vi "ex_readSimpleFile.vi"(5 "first time":bool, 6 "Path":path, 7 "number of lines (all:-1)":i32=-1, 8 "error in":errorcluster, 9 "Generic Header In":string[](array[string]), 10 "string in":string, 11 "Generic Params":T2) -> (0 "error out":errorcluster, 1 "Generic Header Out":string[](array[string]), 2 "string remainder":string, 3 "Signals":waveform(dbl)[](array[waveform]), 4 "EOF":bool)   [LabVIEW 2020]
uses:
  <vilib>/express/express input/ExFileReadBlock.llb/ex_ReadFileGenericParams.ctl
  <vilib>/express/express shared/transition.llb/ex_WaveformAttribs.ctl
  <vilib>/express/express shared/transition.llb/Build Exp Wvfrm (Wvfrm).vi
panel:
  in  "Express Waveform Attributes":T1 {"Timestamp" format="%<%X\n%x>T"; "Start Timestamp" format="%<%X\n%x>T"}
  in  "Array":string[](array[string])
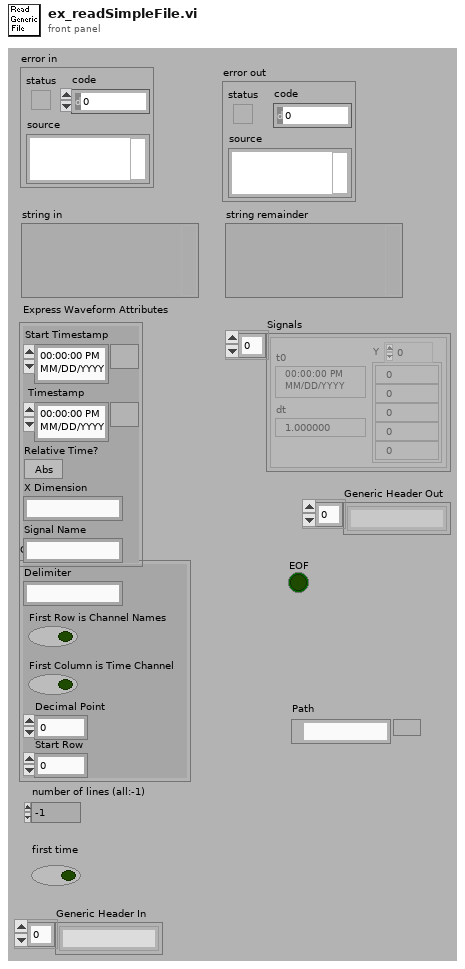
[diagram p1: front panel]
types:
  T1 = typedef "ex_WaveformAttribs.ctl" = cluster{"Start Timestamp":timestamp, "Timestamp":timestamp, "Relative Time?":bool, "X Dimension":string, "Signal Name":string}
  T2 = typedef "ex_ReadFileGenericParams.ctl" = cluster{"Delimiter":string, "First Row is Channel Names":bool, "First Column is Time Channel":bool, "Decimal Point":i32, "Start Row":i32}
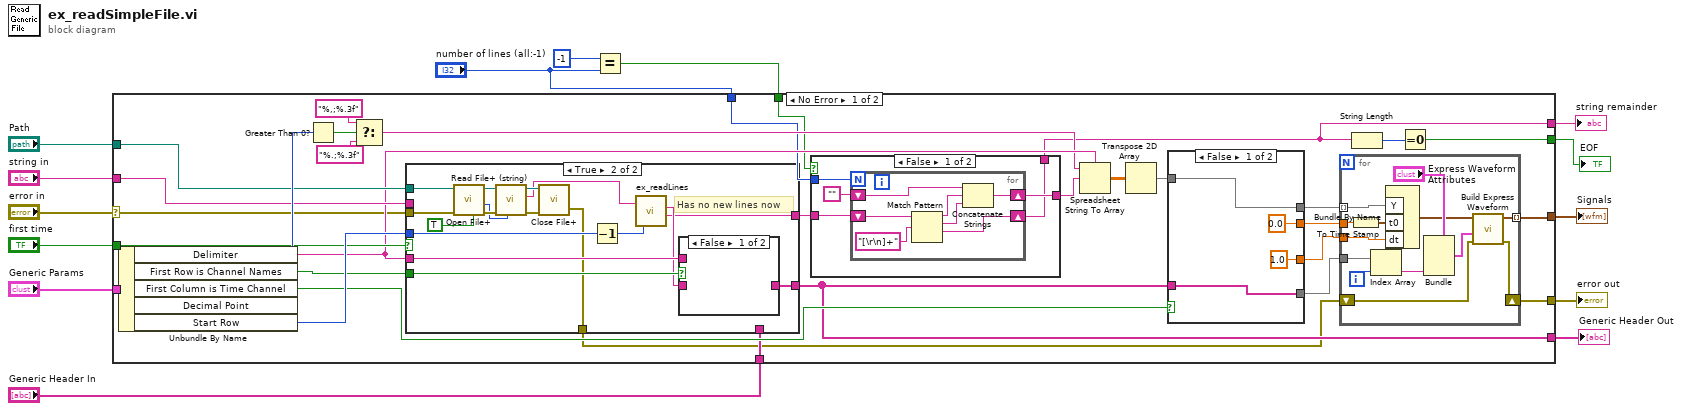
[diagram p0: block diagram]
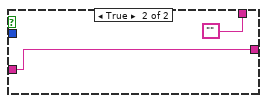
[diagram p2: hidden frame]
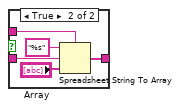
[diagram p5: hidden frame]
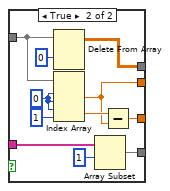
[diagram p6: hidden frame]
diagram:
  n1 = Equal?(x=-1 ("y"), y="number of lines (all:-1)") -> (x = y?=w5:bool)
  n2 = case shown="No Error" "error in" {
    selector: "error in" -> [w16 w117]
    tunnel: [w31 w117] -> w14
    tunnel: [w46 _] -> w13
    tunnel: "Generic Params" -> [w45 _]
    tunnel: "string in" -> [w32 _]
    tunnel: "first time" -> [w30 _]
    tunnel: [w29 _] -> w8
    tunnel: "Generic Header In" -> [w28 _]
    tunnel: [w17 _] -> w6
    tunnel: w5 -> [w20 _]
    tunnel: "number of lines (all:-1)" -> [w21 _]
    tunnel: [w26 _] -> w2
    tunnel: "Path" -> [w25 _]
    frame No Error {
      n3 = Unbundle By Name(w45) -> ("Delimiter"=w23:string, "First Row is Channel Names"=w42:bool, "First Column is Time Channel"=w41:bool, "Decimal Point"=w44:i32, "Start Row"=w43:i32)
      n4 = Greater Than 0?(x=w44) -> (x > 0?=w38:bool)
      n5 = Select(t="%,;%.3f" ("format (%.3f)"), s=w38, f="%.;%.3f" ("format (%.3f)")) -> (s? t:f=w22:string)
      n6 = case shown="True" w30 {
        tunnel: w23 -> [_ w83]
        tunnel: w43 -> [_ w82]
        tunnel: w42 -> [w64 w81]
        tunnel: [w65 w79] -> w19
        tunnel: [w63 w78] -> w29
        tunnel: w32 -> [w65 _]
        tunnel: w28 -> [w62 _]
        tunnel: w25 -> [_ w72]
        tunnel: w16 -> [w61 w68]
        tunnel: [w61 w67] -> w15
        frame False {
          n7 = case shown="False" w64 {
            tunnel: [_ w66] -> w63
            tunnel: w62 -> [_ w66]
            frame False {
            }
            frame True {
            }
          }
        }
        frame True {
          # "Has no new lines now"
          n8 = call <vilib>:"Open File+.vi"("advisory dialog? (display:T)"=TRUE, "error in (not an error)"=w68, "file path (\" \")"=w72) -> ("error out"=w73:errorcluster, "file size (bytes)"=w70:i32, "refnum"=w75:refnum<file>)  [unwired: 4 in, 2 out]
          n9 = call <vilib>:"Read File+ (string).vi"("count"=w70, "error in (no error)"=w73, "refnum"=w75) -> ("error out"=w74:errorcluster, "string"=w71:string, "dup refnum"=w76:refnum<file>)  [unwired: 2 in, 4 out]
          n10 = call <vilib>:"Close File+.vi"("error in (no error)"=w74, "refnum"=w76) -> ("error out"=w67:errorcluster)  [unwired: 5 out]
          n11 = Decrement(x=w82) -> (x-1=w77:i32)
          n12 = call <vilib>:"ex_readLines.vi"("line string"=w71, "# Lines to Skip"=w77) -> ("Channel Names"=w80:string, "Data"=w79:string)  [unwired: 2 out]
          n13 = case shown="False" w81 {
            tunnel: w80 -> [_ w88]
            tunnel: w83 -> [_ w86]
            tunnel: [_ w84] -> w78
            frame False {
            }
            frame True {
              n14 = Spreadsheet String To Array(delimiter (Tab)=w86, format string="%s", spreadsheet string=w88, array type (2D Dbl)="Array") -> (array=w84:string[])
            }
          }
        }
      }
      n15 = case shown="False" w20 {
        tunnel: w21 -> [w51 _]
        tunnel: w19 -> [w50 w60]
        tunnel: [w48 w60] -> w18
        tunnel: [w47 ""] -> w17
        frame False {
          n16 = for {
            N: w51 -> [_]
            shift-right: [w52] -> w47
            shift-left: w50 -> [w58]
            shift-right: [w53] -> w48
            shift-left: "" -> [w56]
            n17 = Match Pattern(string=w58, regular expression="[\r\n]+") -> (before substring=w55:string, match substring=w54:string, after substring=w52:string)  [unwired: 2 out]
            n18 = Concatenate Strings(w56, w55, w54) -> (w53:string)
          }
        }
        frame True {
        }
      }
      n19 = Spreadsheet String To Array(delimiter (Tab)=w23, format string=w22, spreadsheet string=w18) -> (array=w24:dbl[][])  [unwired: 1 out]
      n20 = Transpose 2D Array(2D array=w24) -> (transposed array=w37:dbl[][])
      n21 = case shown="False" w41 {
        tunnel: w37 -> [w92 w101]
        tunnel: [w92 w102] -> w36
        tunnel: [1.0 w99] -> w35
        tunnel: [0.0 w98] -> w34
        tunnel: w29 -> [w89 w95]
        tunnel: [w89 w93] -> w33
        frame False {
        }
        frame True {
          w97 = 0 ("index (row)")
          n22 = Delete From Array(array=w101, index (row)=0) -> (array with subset deleted=w102:dbl[][])  [unwired: 2 in, 1 out]
          n23 = Index Array(array=w101, index (row) #1=w97, index (col) #1=w97, index (row) #2=w97, index (col) #2=1 ("index (row)")) -> (element #1=w98:dbl, element #2=w100:dbl)
          n24 = Array Subset(array=w95, index=1) -> (w93:string[])  [unwired: 1 in]
          n25 = Subtract(x=w100, y=w98) -> (x-y=w99:dbl)
        }
      }
      n26 = for {
        tunnel: [w109] -> w46 mode=indexing
        tunnel: w36 -> [w116] mode=indexing
        tunnel: w33 -> [w115]
        tunnel: w35 -> [w108]
        tunnel: w34 -> [w106]
        shift-right: [w104] -> w31
        shift-left: w15 -> [w105]
        i -> [w114]
        n27 = To Time Stamp(1:w106) -> (0:w107:timestamp)
        n28 = Index Array(array=w115, index=w114) -> (element=w112:string)
        n29 = Bundle By Name("Y"=w116, "t0"=w107, "dt"=w108) -> (w110:waveform(dbl))  [unwired: 1 out]
        n30 = Bundle(cluster="Express Waveform Attributes", "Signal Name"=w112) -> (w111:T1)  [unwired: 4 out]
        n31 = call-poly <vilib>:"Build Express Waveform.vi"("error in (no error)"=w105, "Express Waveform Attributes"=w111, "Waveform"=w110) -> ("error out"=w104:errorcluster, "Waveform"=w109:waveform(dbl))  [unwired: 7 out]
      }
      n32 = String Length(string=w17) -> (length=w27:i32)
      n33 = Equal To 0?(x=w27) -> (x = 0?=w26:bool)
    }
    frame Error {
    }
  }
  "error out" <- w14
  "Signals" <- w13
  "string remainder" <- w6
  "Generic Header Out" <- w8
  "EOF" <- w2
